vi "LIA_read_dual_sens.vi"(8 "error in (no error)":errorcluster, 11 "VISA session (in)":refnum<visa-resource-name>) -> (0 "error out":errorcluster, 2 "Range dual mode Out":u8 step=1, 3 "VISA session (out)":refnum<visa-resource-name>)   [LabVIEW 2019]
uses:
  Equipment/LIA7230/SR7230LV8.llb/SR7230 VISA Write/Read.vi
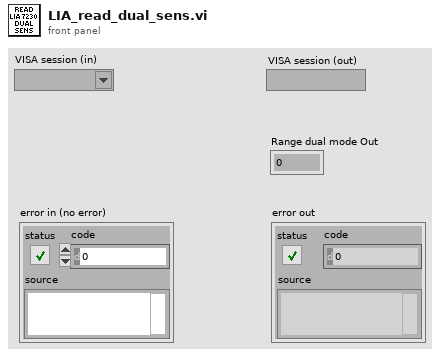
[diagram p1: front panel]
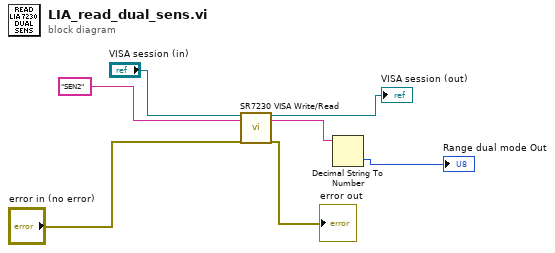
[diagram p0: block diagram]
diagram:
  n1 = call "SR7230 VISA Write/Read.vi"("VISA session (for class)"="VISA session (in)", "Write Command String"="SEN2" ("f"), "error in (no error)"="error in (no error)") -> ("VISA session"=→"VISA session (out)":refnum<visa-resource-name>, "Response 1"=w5:string, "error out"=→"error out":errorcluster)  [unwired: 4 in, 10 out]
  n2 = Decimal String To Number(string=w5) -> (number=→"Range dual mode Out":i32)  [unwired: 2 in, 1 out]
